vi "2283_logicaDeSwitch.vi"(1 "Input":bool) -> (0 "Output":bool)   [LabVIEW 2014]
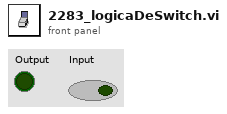
[diagram p1: front panel]
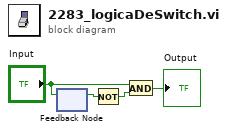
[diagram p0: block diagram]
diagram:
  n1 = feedback #1() -> (w3:bool)  [unwired: 1 in]
  n2 = feedback-in #1("Input") -> ()
  n3 = Not(x=w3) -> (.not. x?=w2:bool)
  n4 = And(x="Input", y=w2) -> (x .and. y?=→"Output":bool)
